vi "Transpose Linear Coordinates.vi"(8 "error in (no error)":errorcluster, 9 "Dim 1":sgl, 10 "Dim 0":sgl, 11 "Transposed Linear Coordinates":refnum<class "2D Array f32.lvclass">) -> (0 "error out":errorcluster, 3 "Corrected Linear Coordinates":refnum<class "2D Array f32.lvclass">)   [LabVIEW 2024, in "G2CPU Line Profile.lvlib"]
uses:
  G2CPU Line Profile.lvlib
  <vilib>/Natan Biesmans/G2CPU GPU and CPU HPC Toolkit/G2CPU Libraries/Arrays/2DArray/f32/2D Array f32.lvclass
  C:/Program Files/National Instruments/LabVIEW 2025/vi.lib/Natan Biesmans/G2CPU GPU and CPU HPC Toolkit/G2CPU Libraries/Arrays/Array/Array Prototype.lvclass
  08227470-474a-4981-913e-10492f30d009.vi
  f811380b-d319-451f-96e9-64ca6ad9fc86.vi
  8480a7f2-12d0-4fb9-879e-d86aedec7196.vi
  8dedf08d-1ef7-468d-bcc1-e9b02c4e024f.vi
  7f93758b-77ec-40e5-ad19-6efb6668d24e.vi
  08227470-474a-4981-913e-10492f30d009.vi/9d769ba4-bbb4-4eb6-9175-95d7d139327c.vi
  08227470-474a-4981-913e-10492f30d009.vi/8bfea9e7-a130-4d69-b32e-15c58d17157f.vi
  08227470-474a-4981-913e-10492f30d009.vi/25f1b8bb-c437-45f4-b6eb-f3e32cc20aa5.vi
  08227470-474a-4981-913e-10492f30d009.vi/309f54b5-9a40-4a1d-900d-2d620fefb202.vi
  f811380b-d319-451f-96e9-64ca6ad9fc86.vi/bb516b05-0a1d-45df-9cb0-c772dcc1833e.vi
  f811380b-d319-451f-96e9-64ca6ad9fc86.vi/2071ba82-ee09-44c2-9784-3e752811cb07.vi
  f811380b-d319-451f-96e9-64ca6ad9fc86.vi/c68a08d6-cad3-47fe-810c-4c138e8e5bf7.vi
  f811380b-d319-451f-96e9-64ca6ad9fc86.vi/599fcc89-82aa-4e20-b9df-949478d910a7.vi
  8480a7f2-12d0-4fb9-879e-d86aedec7196.vi/4181b2af-0669-475f-8228-b34a8d51a6f4.vi
  8dedf08d-1ef7-468d-bcc1-e9b02c4e024f.vi/6197f869-f6d4-49b3-9b2c-cc979b422c2e.vi
  8dedf08d-1ef7-468d-bcc1-e9b02c4e024f.vi/a7e86dbb-b4c0-485c-89c5-522e60ee265c.vi
  7f93758b-77ec-40e5-ad19-6efb6668d24e.vi/5793b77b-c002-4ebf-9075-685617c95341.vi
  7f93758b-77ec-40e5-ad19-6efb6668d24e.vi/2ed3ef86-c00d-4d71-b84c-20267a6dfcf9.vi
  08227470-474a-4981-913e-10492f30d009.vi/8bfea9e7-a130-4d69-b32e-15c58d17157f.vi/3587aa3f-97a0-4074-a424-c31da557ec96.vi
  08227470-474a-4981-913e-10492f30d009.vi/8bfea9e7-a130-4d69-b32e-15c58d17157f.vi/6058dca8-195d-4566-b47b-6d6a1c5af61f.vi
  08227470-474a-4981-913e-10492f30d009.vi/309f54b5-9a40-4a1d-900d-2d620fefb202.vi/730f6c57-5c0b-4ee9-b61e-75067b25222b.vi
  08227470-474a-4981-913e-10492f30d009.vi/309f54b5-9a40-4a1d-900d-2d620fefb202.vi/096b8799-7810-404e-baca-ba9279cec4bd.vi
  08227470-474a-4981-913e-10492f30d009.vi/309f54b5-9a40-4a1d-900d-2d620fefb202.vi/0f1a5a47-bcc5-4796-ac31-8dfcfbc0d7d1.vi
  08227470-474a-4981-913e-10492f30d009.vi/309f54b5-9a40-4a1d-900d-2d620fefb202.vi/89f12e17-3330-4b72-ad8f-8dd636660732.vi
  f811380b-d319-451f-96e9-64ca6ad9fc86.vi/bb516b05-0a1d-45df-9cb0-c772dcc1833e.vi/46771f49-eb1d-473b-8e81-f516cef50a4e.vi
  f811380b-d319-451f-96e9-64ca6ad9fc86.vi/bb516b05-0a1d-45df-9cb0-c772dcc1833e.vi/dc76f8e4-64fa-456a-8549-7a4b6936c4c9.vi
  f811380b-d319-451f-96e9-64ca6ad9fc86.vi/bb516b05-0a1d-45df-9cb0-c772dcc1833e.vi/7e60ddfb-e748-4c0c-85da-e395a1b7978d.vi
  f811380b-d319-451f-96e9-64ca6ad9fc86.vi/bb516b05-0a1d-45df-9cb0-c772dcc1833e.vi/d2eceff7-f641-4ce4-acfa-e9e293a3c877.vi
  f811380b-d319-451f-96e9-64ca6ad9fc86.vi/bb516b05-0a1d-45df-9cb0-c772dcc1833e.vi/b737122b-4036-448b-abd3-e2701355e828.vi
  f811380b-d319-451f-96e9-64ca6ad9fc86.vi/2071ba82-ee09-44c2-9784-3e752811cb07.vi/a578f522-3460-4434-be98-bad896664269.vi
  f811380b-d319-451f-96e9-64ca6ad9fc86.vi/c68a08d6-cad3-47fe-810c-4c138e8e5bf7.vi/e7247370-a01f-465a-ac0e-4dfefcb1bb87.vi
  f811380b-d319-451f-96e9-64ca6ad9fc86.vi/c68a08d6-cad3-47fe-810c-4c138e8e5bf7.vi/345e91f0-9a5e-4de4-af9c-133346717e4a.vi
  8dedf08d-1ef7-468d-bcc1-e9b02c4e024f.vi/6197f869-f6d4-49b3-9b2c-cc979b422c2e.vi/87b81512-7a6a-4bb0-93b2-4564eba18751.vi
  8dedf08d-1ef7-468d-bcc1-e9b02c4e024f.vi/6197f869-f6d4-49b3-9b2c-cc979b422c2e.vi/3b85cfcd-f2e7-425d-bf63-d84251333cff.vi
  8dedf08d-1ef7-468d-bcc1-e9b02c4e024f.vi/6197f869-f6d4-49b3-9b2c-cc979b422c2e.vi/bdde7ba0-fc5a-4512-a8ec-1695e5fcee25.vi
  8dedf08d-1ef7-468d-bcc1-e9b02c4e024f.vi/6197f869-f6d4-49b3-9b2c-cc979b422c2e.vi/3e802c67-fb96-46a3-ae13-4994a8508b4f.vi
  8dedf08d-1ef7-468d-bcc1-e9b02c4e024f.vi/6197f869-f6d4-49b3-9b2c-cc979b422c2e.vi/5a50fc67-79e7-4972-80c2-92243cd53dd4.vi
  8dedf08d-1ef7-468d-bcc1-e9b02c4e024f.vi/a7e86dbb-b4c0-485c-89c5-522e60ee265c.vi/730f6c57-5c0b-4ee9-b61e-75067b25222b.vi
  8dedf08d-1ef7-468d-bcc1-e9b02c4e024f.vi/a7e86dbb-b4c0-485c-89c5-522e60ee265c.vi/096b8799-7810-404e-baca-ba9279cec4bd.vi
  8dedf08d-1ef7-468d-bcc1-e9b02c4e024f.vi/a7e86dbb-b4c0-485c-89c5-522e60ee265c.vi/0f1a5a47-bcc5-4796-ac31-8dfcfbc0d7d1.vi
  8dedf08d-1ef7-468d-bcc1-e9b02c4e024f.vi/a7e86dbb-b4c0-485c-89c5-522e60ee265c.vi/89f12e17-3330-4b72-ad8f-8dd636660732.vi
  7f93758b-77ec-40e5-ad19-6efb6668d24e.vi/5793b77b-c002-4ebf-9075-685617c95341.vi/3e802c67-fb96-46a3-ae13-4994a8508b4f.vi
  7f93758b-77ec-40e5-ad19-6efb6668d24e.vi/5793b77b-c002-4ebf-9075-685617c95341.vi/5a50fc67-79e7-4972-80c2-92243cd53dd4.vi
  7f93758b-77ec-40e5-ad19-6efb6668d24e.vi/2ed3ef86-c00d-4d71-b84c-20267a6dfcf9.vi/730f6c57-5c0b-4ee9-b61e-75067b25222b.vi
  7f93758b-77ec-40e5-ad19-6efb6668d24e.vi/2ed3ef86-c00d-4d71-b84c-20267a6dfcf9.vi/096b8799-7810-404e-baca-ba9279cec4bd.vi
  7f93758b-77ec-40e5-ad19-6efb6668d24e.vi/2ed3ef86-c00d-4d71-b84c-20267a6dfcf9.vi/0f1a5a47-bcc5-4796-ac31-8dfcfbc0d7d1.vi
  7f93758b-77ec-40e5-ad19-6efb6668d24e.vi/2ed3ef86-c00d-4d71-b84c-20267a6dfcf9.vi/89f12e17-3330-4b72-ad8f-8dd636660732.vi
  08227470-474a-4981-913e-10492f30d009.vi/8bfea9e7-a130-4d69-b32e-15c58d17157f.vi/6058dca8-195d-4566-b47b-6d6a1c5af61f.vi/77c7badc-ed81-4514-99c1-20d37f4e5ecc.vi
  08227470-474a-4981-913e-10492f30d009.vi/8bfea9e7-a130-4d69-b32e-15c58d17157f.vi/6058dca8-195d-4566-b47b-6d6a1c5af61f.vi/eb76fa01-6782-47b4-b34f-9eb474c9cc78.vi
  f811380b-d319-451f-96e9-64ca6ad9fc86.vi/bb516b05-0a1d-45df-9cb0-c772dcc1833e.vi/dc76f8e4-64fa-456a-8549-7a4b6936c4c9.vi/2c12aba4-aacf-4d7a-adbe-039f6155a93e.vi
  f811380b-d319-451f-96e9-64ca6ad9fc86.vi/bb516b05-0a1d-45df-9cb0-c772dcc1833e.vi/dc76f8e4-64fa-456a-8549-7a4b6936c4c9.vi/f38cccb2-46f6-49f0-a8d6-9da0c88ff6f3.vi
  f811380b-d319-451f-96e9-64ca6ad9fc86.vi/bb516b05-0a1d-45df-9cb0-c772dcc1833e.vi/dc76f8e4-64fa-456a-8549-7a4b6936c4c9.vi/bdde7ba0-fc5a-4512-a8ec-1695e5fcee25.vi
  f811380b-d319-451f-96e9-64ca6ad9fc86.vi/bb516b05-0a1d-45df-9cb0-c772dcc1833e.vi/dc76f8e4-64fa-456a-8549-7a4b6936c4c9.vi/3e802c67-fb96-46a3-ae13-4994a8508b4f.vi
  f811380b-d319-451f-96e9-64ca6ad9fc86.vi/bb516b05-0a1d-45df-9cb0-c772dcc1833e.vi/dc76f8e4-64fa-456a-8549-7a4b6936c4c9.vi/5a50fc67-79e7-4972-80c2-92243cd53dd4.vi
  8dedf08d-1ef7-468d-bcc1-e9b02c4e024f.vi/6197f869-f6d4-49b3-9b2c-cc979b422c2e.vi/3e802c67-fb96-46a3-ae13-4994a8508b4f.vi/1b7cf390-2ae0-48f3-9bce-03c57eed6ee8.vi
  f811380b-d319-451f-96e9-64ca6ad9fc86.vi/bb516b05-0a1d-45df-9cb0-c772dcc1833e.vi/dc76f8e4-64fa-456a-8549-7a4b6936c4c9.vi/5a50fc67-79e7-4972-80c2-92243cd53dd4.vi/1b7cf390-2ae0-48f3-9bce-03c57eed6ee8.vi
  <vilib>/Natan Biesmans/G2CPU GPU and CPU HPC Toolkit/G2CPU Libraries/Arrays/1DArray/f32/1D Array f32.lvclass
  <vilib>/Natan Biesmans/G2CPU GPU and CPU HPC Toolkit/ArrayFire Driver/VIs/Run as Multi Device.vi
  <vilib>/Natan Biesmans/G2CPU GPU and CPU HPC Toolkit/G2CPU Libraries/Arrays/Array/G2CPU Get Array Pointer.vi
  <vilib>/Natan Biesmans/G2CPU GPU and CPU HPC Toolkit/ArrayFire Driver/VIs/iszero.vi
  <vilib>/Natan Biesmans/G2CPU GPU and CPU HPC Toolkit/ArrayFire Driver/VIs/sub.vi
  <vilib>/Natan Biesmans/G2CPU GPU and CPU HPC Toolkit/ArrayFire Driver/VIs/release array.vi
  <vilib>/Natan Biesmans/G2CPU GPU and CPU HPC Toolkit/G2CPU Libraries/Manage Environment/Find AF DLL.vi
  <vilib>/Natan Biesmans/G2CPU GPU and CPU HPC Toolkit/ArrayFire Driver/subvi/Error Converter (ErrCode or Status).vi
  <vilib>/Natan Biesmans/G2CPU GPU and CPU HPC Toolkit/ArrayFire Driver/VIs/cast.vi
  <vilib>/Natan Biesmans/G2CPU GPU and CPU HPC Toolkit/ArrayFire Driver/VIs/add.vi
  <vilib>/Natan Biesmans/G2CPU GPU and CPU HPC Toolkit/G2CPU Libraries/Arrays/Array/G2CPU Set Array Pointer.vi
  <vilib>/Natan Biesmans/G2CPU GPU and CPU HPC Toolkit/G2CPU Libraries/Arrays/SubVI/Lock Arrays.vi
  <vilib>/Natan Biesmans/G2CPU GPU and CPU HPC Toolkit/G2CPU Libraries/Arrays/SubVI/is 2D.vi
  <vilib>/Natan Biesmans/G2CPU GPU and CPU HPC Toolkit/ArrayFire Driver/VIs/mod.vi
  <vilib>/Natan Biesmans/G2CPU GPU and CPU HPC Toolkit/G2CPU Libraries/Arrays/Array/G2CPU Unlock Array.vi
  <vilib>/Natan Biesmans/G2CPU GPU and CPU HPC Toolkit/G2CPU Libraries/Arrays/Array/G2CPU Release Array.vi
  <vilib>/Natan Biesmans/G2CPU GPU and CPU HPC Toolkit/ArrayFire Driver/VIs/div.vi
  <vilib>/Natan Biesmans/G2CPU GPU and CPU HPC Toolkit/G2CPU Libraries/Arrays/Array/G2CPU Lock Array.vi
  <vilib>/Natan Biesmans/G2CPU GPU and CPU HPC Toolkit/ArrayFire Driver/VIs/trunc.vi
  <vilib>/Natan Biesmans/G2CPU GPU and CPU HPC Toolkit/ArrayFire Driver/VIs/round.vi
  <vilib>/Natan Biesmans/G2CPU GPU and CPU HPC Toolkit/ArrayFire Driver/VIs/mul.vi
  <vilib>/Natan Biesmans/G2CPU GPU and CPU HPC Toolkit/G2CPU Libraries/Arrays/Array/Array Prototype.lvclass
  <vilib>/Natan Biesmans/G2CPU GPU and CPU HPC Toolkit/G2CPU Libraries/Arrays/2DArray/2D Array Prototype.lvclass
  <vilib>/Natan Biesmans/G2CPU GPU and CPU HPC Toolkit/G2CPU Libraries/Arrays/DataTypes/f32/f32.lvclass
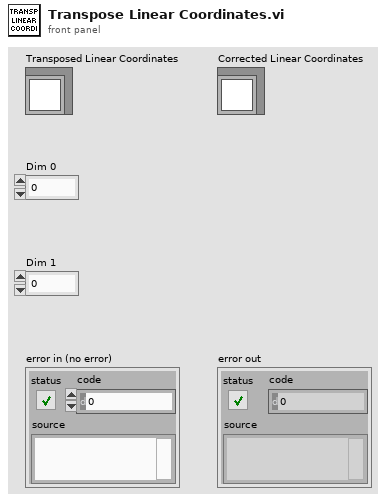
[diagram p1: front panel]
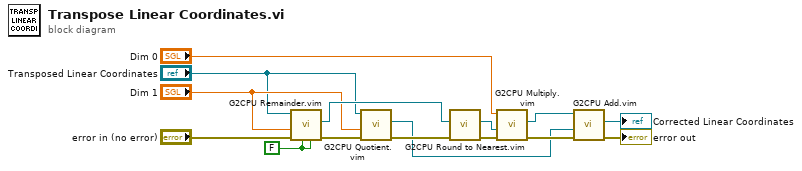
[diagram p0: block diagram]
diagram:
  w4 = FALSE ("Auto Release lhs (Enabled)")
  n1 = call "G2CPU Remainder.vim"("Auto Release rhs (Enabled)"=w4, "Auto Release lhs (Enabled)"=w4, "error in (no error)"="error in (no error)", "Array rhs"="Dim 1", "Array lhs"="Transposed Linear Coordinates") -> ("error out"=w3:errorcluster, "Array Result"=w8:refnum<class "2D Array f32.lvclass">)  [unwired: 5 in]
  n2 = call "G2CPU Quotient.vim"("error in (no error)"=w3, "Array rhs"="Dim 1", "Array lhs"="Transposed Linear Coordinates") -> ("error out"=w12:errorcluster, "Array Result"=w7:refnum<class "2D Array f32.lvclass">)  [unwired: 7 in]
  n3 = call "G2CPU Round to Nearest.vim"("error in (no error)"=w12, "Array in"=w8) -> ("error out"=w13:errorcluster, "Array Result"=w9:refnum<class "2D Array f32.lvclass">)  [unwired: 8 in]
  n4 = call "G2CPU Multiply.vim"("error in (no error)"=w13, "Array rhs"=w9, "Array lhs"="Dim 0") -> ("error out"=w14:errorcluster, "Array Result"=w6:refnum<class "2D Array f32.lvclass">)  [unwired: 7 in]
  n5 = call "G2CPU Add.vim"("error in (no error)"=w14, "Array rhs"=w7, "Array lhs"=w6) -> ("error out"=→"error out":errorcluster, "Array Result"=→"Corrected Linear Coordinates":refnum<class "2D Array f32.lvclass">)  [unwired: 7 in]
